vi "set_S34CON.vi"(8 "error in (no error)":errorcluster caption="错误输入（无错误）", 9 "S34CON寄存器和P4设置":T1={"TRUE: P4 出低电平; FALSE: P4 出高电平。"=FALSE, "P4输出关联的事件代码"=0, "S3传感器上升沿绑定动作"=0, "S3传感器下降沿绑定动作"=1, "当发生堵转时动作"=1} {"当发生堵转时动作" items=["无动作，无状态通知", "无动作，有通知", "负向连续运行", "减速直到停止", "紧急停止", "负向相对位移控制", "绝对位置清零", "绝对位置清零+相对位移控制", "", "换向相对位移控制", "正向连续运行", "绝对位置清零+减速直到停止", "绝对位置清零+紧急停止", "正向相对位移控制", "换向连续运行", "脱机"]; "P4输出关联的事件代码" items=["无动作，无状态通知", "电机转动，P4=指定电平；反之，P4相反", "电机正转，P4=指定电平；反之，P4相反", "位移大于等于0，P4=指定电平；反之，P4相反"]; "S3传感器下降沿绑定动作" items=["无动作，无状态通知"=0, "无动作，有通知"=1, "负向连续运行"=2, "减速直到停止"=3, "紧急停止"=4, "负向相对位移控制"=5, "绝对位置清零"=6, "绝对位置清零+相对位移控制"=7, "换向相对位移控制"=9, "正向连续运行"=10, "绝对位置清零+减速直到停止"=11, "绝对位置清零+紧急停止"=12, "正向相对位移控制"=13, "换向连续运行"=14, "脱机"=15]; "S3传感器上升沿绑定动作" items=["无动作，无状态通知"=0, "无动作，有通知"=1, "负向连续运行"=2, "减速直到停止"=3, "紧急停止"=4, "负向相对位移控制"=5, "绝对位置清零"=6, "绝对位置清零+相对位移控制"=7, "换向相对位移控制"=9, "正向连续运行"=10, "绝对位置清零+减速直到停止"=11, "绝对位置清零+紧急停止"=12, "正向相对位移控制"=13, "换向连续运行"=14, "脱机"=15]}, 11 "StepMotor输入":refnum<class "StepMotor.lvclass">) -> (0 "error out":errorcluster caption="错误输出", 3 "StepMotor输出":refnum<class "StepMotor.lvclass">)   [LabVIEW 2016, in "MotionControl.lvlib" / "StepMotor.lvclass"]
uses:
  <userlib>/MotionControl/StepMotor/StepMotor.lvclass
  <userlib>/MotionControl/StepMotor/S34CON.ctl
  <userlib>/MotionControl/StepMotor/StepMotor.lvclass/StepMotor.ctl
  <userlib>/UISimCanFunc_wrapper/UISimCanFunc_wrapper.lvlib
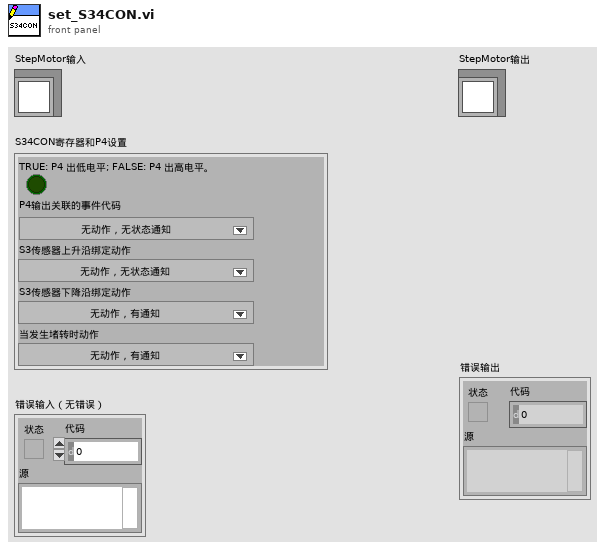
[diagram p1: front panel]
types:
  T1 = typedef "MotionControl.lvlib/StepMotor.lvclass/S34CON.ctl" = cluster{"TRUE: P4 出低电平; FALSE: P4 出高电平。":bool, "P4输出关联的事件代码":u32, "S3传感器上升沿绑定动作":u32, "S3传感器下降沿绑定动作":u32, "当发生堵转时动作":u32}
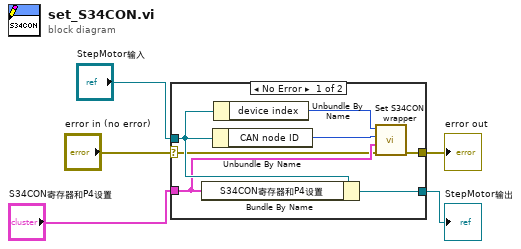
[diagram p0: block diagram]
diagram:
  n1 = case shown="No Error" "error in (no error)" {
    selector: "error in (no error)" -> [w7 w13]
    tunnel: [w6 w13] -> w4
    tunnel: [w12 w14] -> w2
    tunnel: "StepMotor输入" -> [w11 w14]
    tunnel: "S34CON寄存器和P4设置" -> [w8 _]
    frame No Error {
      n2 = Bundle By Name(cluster=w11, "S34CON寄存器和P4设置"=w8) -> (w12:refnum<class "StepMotor.lvclass">)
      n3 = Unbundle By Name(w11) -> ("CAN node ID"=w9:u32)
      n4 = Unbundle By Name(w11) -> ("device index"=w10:u32)
      n5 = call <userlib>:"Set S34CON wrapper.vi"("error in (no error)"=w7, "S34CON In"=w8, "dwCanNodeId"=w9, "dwDevIndex"=w10) -> ("error out"=w6:errorcluster)  [unwired: 5 in, 2 out]
    }
    frame Error {
    }
  }
  "error out" <- w4
  "StepMotor输出" <- w2
